vi "niScope Configure Trigger Software.vi"(0 "instrument handle":refnum<k15>, 11 "error in":errorcluster, 12 "trigger holdoff":dbl format="%.4f", 13 "trigger delay":dbl format="%.4f") -> (4 "instrument handle out":refnum<k15>, 15 "error out":errorcluster)   [LabVIEW 2011]
doc: "Configures common properties for software triggering. This VI only works in an Initiate/Fetch operation."
uses:
  niScope_32.dll
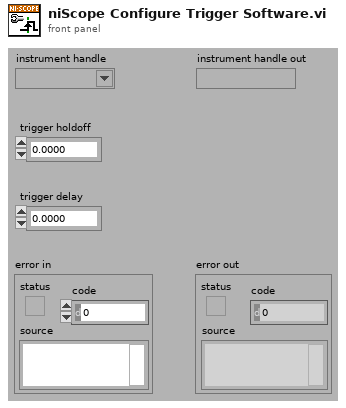
[diagram p1: front panel]
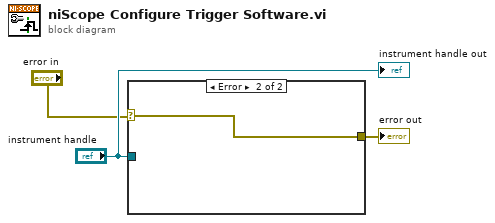
[diagram p0: block diagram]
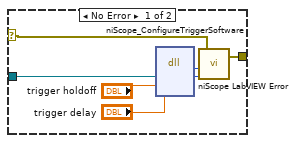
[diagram p2: hidden frame]
diagram:
  n1 = case shown="Error" "error in" {
    selector: "error in" -> [w4 w11]
    tunnel: [w7 w11] -> w3
    tunnel: "instrument handle" -> [w10 _]
    frame No Error {
      n2 = dll-call lib="niScope_*.*" fn="niScope_ConfigureTriggerSoftware"("instrument handle"=w10, "holdoff"="trigger holdoff", "delay"="trigger delay") -> ("status"=w9:i32, "instrument handle"=w8:u32)  [unwired: 5 in, 2 out]
      n3 = call <instrlib>:"niScope LabVIEW Error.vi"("instrument handle"=w8, "niScope error code (0)"=w9, "error in (no error)"=w4) -> ("error out"=w7:errorcluster)  [unwired: 2 in]
    }
    frame Error {
    }
  }
  "error out" <- w3
  "instrument handle out" <- "instrument handle"
